vi "SLL Create Annotation List.vi"(7 "Plot Name":string[](array[string]), 8 "error in (no error)":errorcluster, 9 "Plot Enable?":bool[](array[boolean]), 10 "Annotation Colour":u32[](array[colorbox])=[16777215, 16728642, 982784, 16776704], 11 "Annotation List":T1) -> (0 "error out":errorcluster, 3 "Annotation List Out":T1)   [LabVIEW 2013]
doc: "Copyright © 2005, Soliton Technologies.\nAll rights reserved."
uses:
  Controls/SLL DE Get Plot LV2Global Options.ctl
  <vilib>/Utility/miscctls.llb/LVAnnotationListTypeDef.ctl
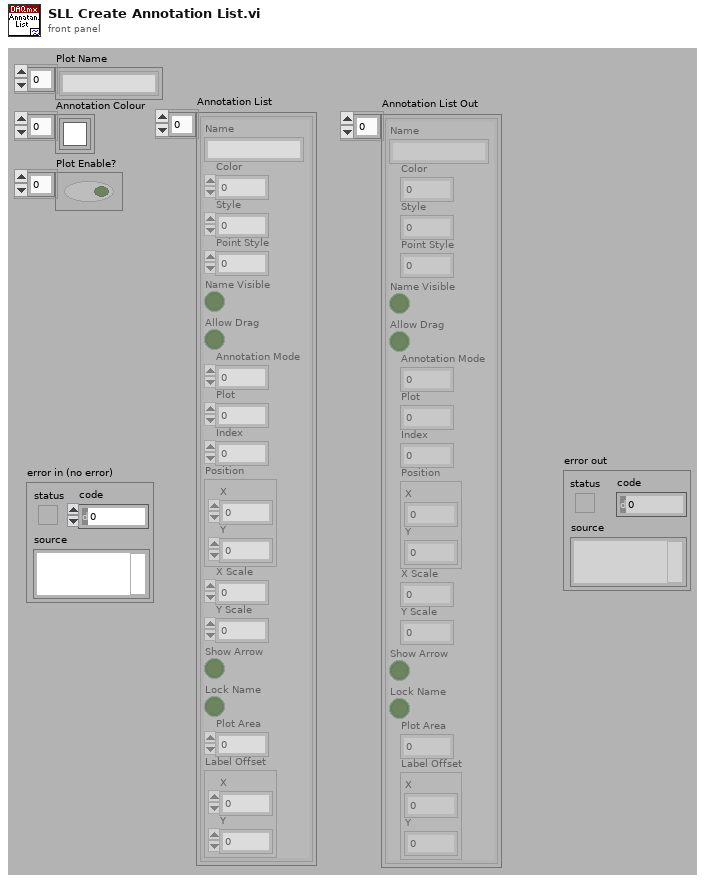
[diagram p1: front panel]
types:
  T1 = typedef "LVAnnotationListTypeDef.ctl" = cluster{"Name":string, "Color":u32, "Style":u8, "Point Style":u8, "Name Visible":bool, "Allow Drag":bool, "Annotation Mode":u32, "Plot":i32, "Index":i32, "Position":cluster{"X":dbl, "Y":dbl}, "X Scale":u32, "Y Scale":u32, "Show Arrow":bool, "Lock Name":bool, "Plot Area":i32, "Label Offset":cluster{"X":dbl, "Y":dbl}}[]
  T2 = typedef "SLL DE Get Plot LV2Global Options.ctl" = enum16{"Init", "Get Plot", "Read Plot"}
  T3 = cluster{"Name":string, "Color":u32, "Style":u8, "Point Style":u8, "Name Visible":bool, "Allow Drag":bool, "Annotation Mode":u32, "Plot":i32, "Index":i32, "Position":cluster{"X":dbl, "Y":dbl}, "X Scale":u32, "Y Scale":u32, "Show Arrow":bool, "Lock Name":bool, "Plot Area":i32, "Label Offset":cluster{"X":dbl, "Y":dbl}}
  T4 = cluster{"Time Scale":sgl[], "Sample Value In":sgl[]}[]
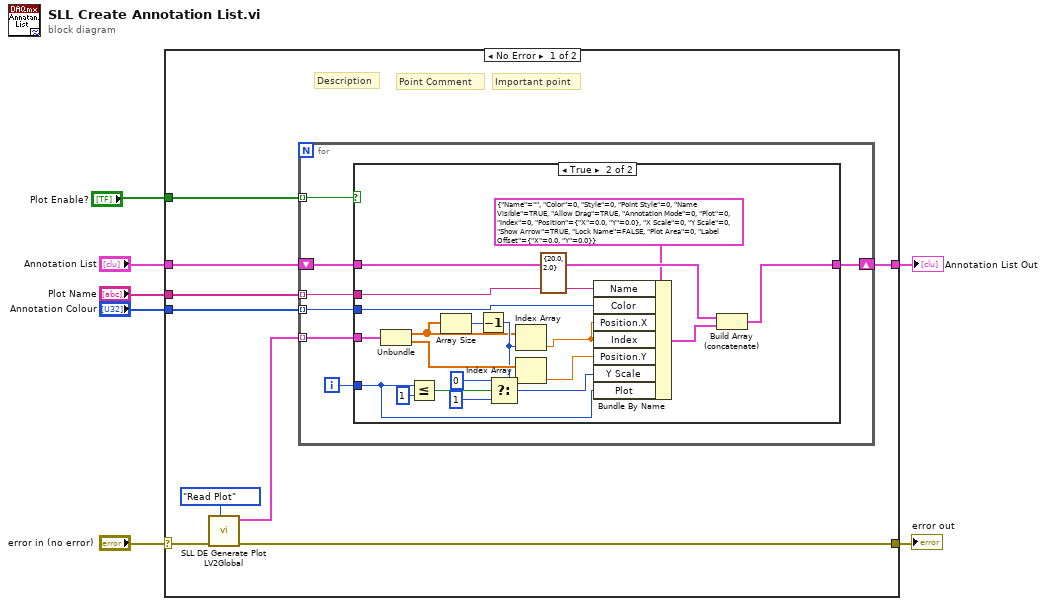
[diagram p0: block diagram]
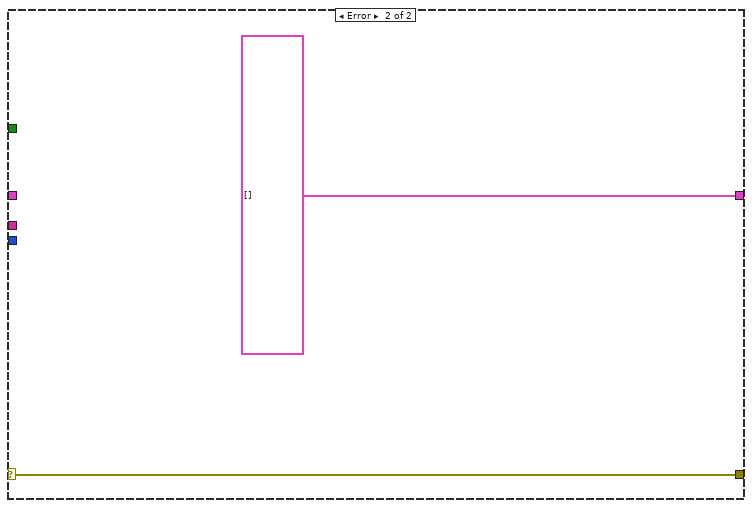
[diagram p3: hidden frame]
diagram:
  n1 = case shown="No Error" "error in (no error)" {
    selector: "error in (no error)" -> [w9 w45]
    tunnel: [w8 w45] -> w6
    tunnel: "Annotation Colour" -> [w14 _]
    tunnel: "Annotation List" -> [w13 _]
    tunnel: "Plot Name" -> [w12 _]
    tunnel: "Plot Enable?" -> [w11 _]
    tunnel: [w10 T1 [] ("Annotation List")] -> w1
    frame No Error {
      # "Point Comment"
      # "Important point"
      # "Description"
      n2 = call "SLL DE Generate Plot LV2Global.vi"("Option"=SLL_DE_Get_Plot_LV2Global_Options."Read Plot", "error in (no error)"=w9) -> ("error IO"=w8:errorcluster, "Plot data array"=w16:T4)  [unwired: 8 in]
      n3 = for {
        tunnel: w11 -> [w22] mode=indexing
        tunnel: w16 -> [w23] mode=indexing
        shift-right: [w20] -> w10
        shift-left: w13 -> [w17]
        tunnel: w14 -> [w19] mode=indexing
        tunnel: w12 -> [w18] mode=indexing
        i -> [w21]
        n4 = case shown="True" w22 {
          tunnel: w23 -> [_ w39]
          tunnel: w21 -> [_ w26]
          tunnel: [w24 w34] -> w20
          tunnel: w19 -> [_ w42]
          tunnel: w18 -> [_ w41]
          tunnel: w17 -> [w24 w40]
          frame False {
          }
          frame True {
            (unwired) cluster{"X":dbl, "Y":dbl} {"X"=20.0, "Y"=2.0} ("Label Offset")
            n5 = Unbundle(w39) -> ("Time Scale"=w27:sgl[], "Sample Value In"=w37:sgl[])
            n6 = Less Or Equal?(x=w26, y=1) -> (x <= y?=w32:bool)
            n7 = Array Size(array=w27) -> (size(s)=w36:i32)
            n8 = Decrement(x=w36) -> (x-1=w35:i32)
            n9 = Select(t=0, s=w32, f=1) -> (s? t:f=w29:i32)
            n10 = Index Array(array=w27, index=w35) -> (element=w25:sgl)
            n11 = Index Array(array=w37, index=w35) -> (element=w38:sgl)
            n12 = Bundle By Name(cluster=T3 {"Name"="", "Color"=0, "Style"=0, "Point Style"=0, "Name Visible"=TRUE, "Allow Drag"=TRUE, "Annotation Mode"=0, "Plot"=0, "Index"=0, "Position"={"X"=0.0, "Y"=0.0}, "X Scale"=0, "Y Scale"=0, "Show Arrow"=TRUE, "Lock Name"=FALSE, "Plot Area"=0, "Label Offset"={"X"=0.0, "Y"=0.0}} ("element"), "Name"=w41, "Color"=w42, "Position.X"=w25, "Index"=w25, "Position.Y"=w38, "Y Scale"=w29, "Plot"=w26) -> (w43:T3)
            n13 = Build Array (concatenate)(w40, w43) -> (w34:T1)
          }
        }
      }
    }
    frame Error {
    }
  }
  "error out" <- w6
  "Annotation List Out" <- w1
